vi "Read Lines.vi"(8 "error in (no error)":errorcluster, 11 "Convert Bool to Velocity configuration in":refnum<class "Convert Bool to Velocity configuration.lvclass">) -> (0 "error out":errorcluster, 2 "Lines":T1(array[cluster]), 3 "Convert Bool to Velocity configuration out":refnum<class "Convert Bool to Velocity configuration.lvclass">)   [LabVIEW 2017, in "Convert Bool to Velocity configuration.lvclass"]
uses:
  Convert Bool to Velocity configuration.lvclass
  <vilib>/NI/Tag Bus Module Framework/channel/TBM channel.lvclass
  Convert Bool to Velocity configuration.lvclass/Convert Bool to Velocity configuration.ctl
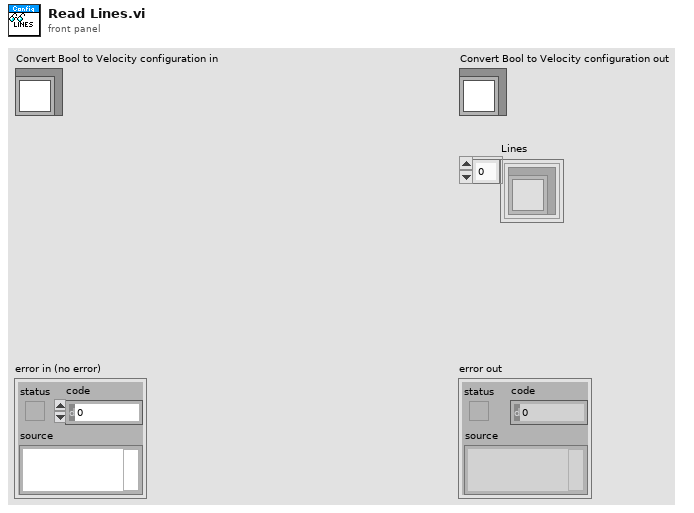
[diagram p1: front panel]
types:
  T1 = cluster{"channel":refnum<class "TBM channel.lvclass">}[]
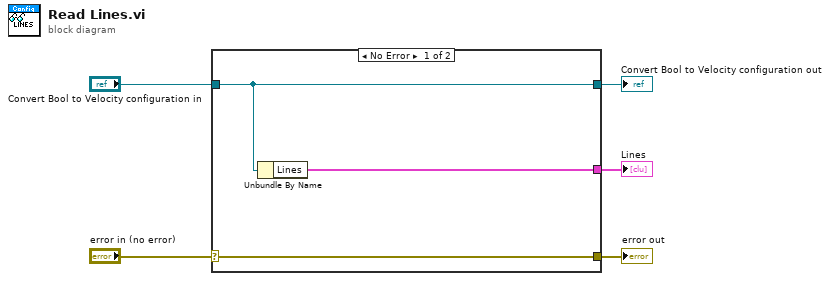
[diagram p0: block diagram]
diagram:
  n1 = case shown="No Error" "error in (no error)" {
    selector: "error in (no error)" -> [w8 w9]
    tunnel: [w8 w9] -> w4
    tunnel: [w7 w10] -> w2
    tunnel: "Convert Bool to Velocity configuration in" -> [w7 w10]
    tunnel: [w6 _] -> w1
    frame No Error {
      n2 = Unbundle By Name(w7) -> ("Lines"=w6:T1)
    }
    frame Error {
    }
  }
  "error out" <- w4
  "Convert Bool to Velocity configuration out" <- w2
  "Lines" <- w1
